vi "coincidenceImagenew.vi"(0 "notes 2":refnum<vi>) -> ()   [LabVIEW 2009]
uses:
  <vilib>/vision/NI_Vision_Development_Module.lvlib
panel:
  in  "notes":string
  in  "RGB/False":bool
  in  "Threshold":cluster{"max":u32, "min":u32}
  out "Photons":u32
  out "Spot No.":u8
  out "Ampel2":cluster{"RED":bool, "YELLOW":bool, "GREEN":bool}
  in  "spotsize (radius pixel)":u16=5 min=1 max=100
  in  "delayed channel":u8 max=7
  in  "length (µs)":dbl=10.0 format="%.2f"
  in  "lateral peaks":u32=2 min=2 max=10 step=2
  in  "center peak (µs)":dbl=0.6 format="%.2f"
  out "coincidence ratio":dbl format="%.2f"
  out "coincidence histogram":T1(graph)
  out "oval coordinates":i32[](array[numeric])
  out "Coordinates":i32[](array[numeric])
  in  "stop":bool
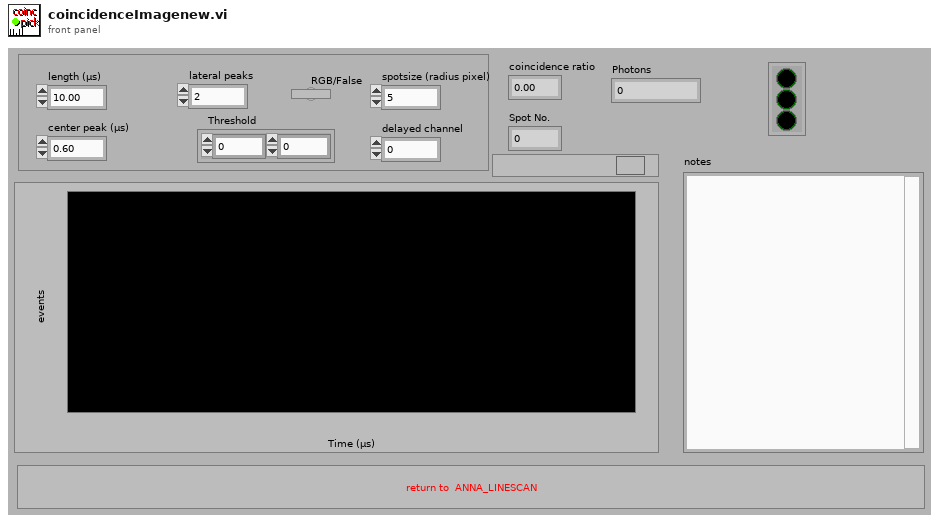
[diagram p1: front panel]
types:
  T1 = cluster{"Origin (ns)":dbl, "Offset (ns)":dbl, u32[]}
  T2 = cluster{"x0":i32, "y0":i32, "x1":i32, "y1":i32, "ovl std":i32[][]}
  T3 = enum16{"read/write", "read-only", "write-only", "write-only (truncate)"}
  T4 = typedef "IMAQ Image.ctl" = refnum<image>
  T5 = cluster{"origin (ns)":dbl, "offset (ns)":dbl, "histogram":u32[]}
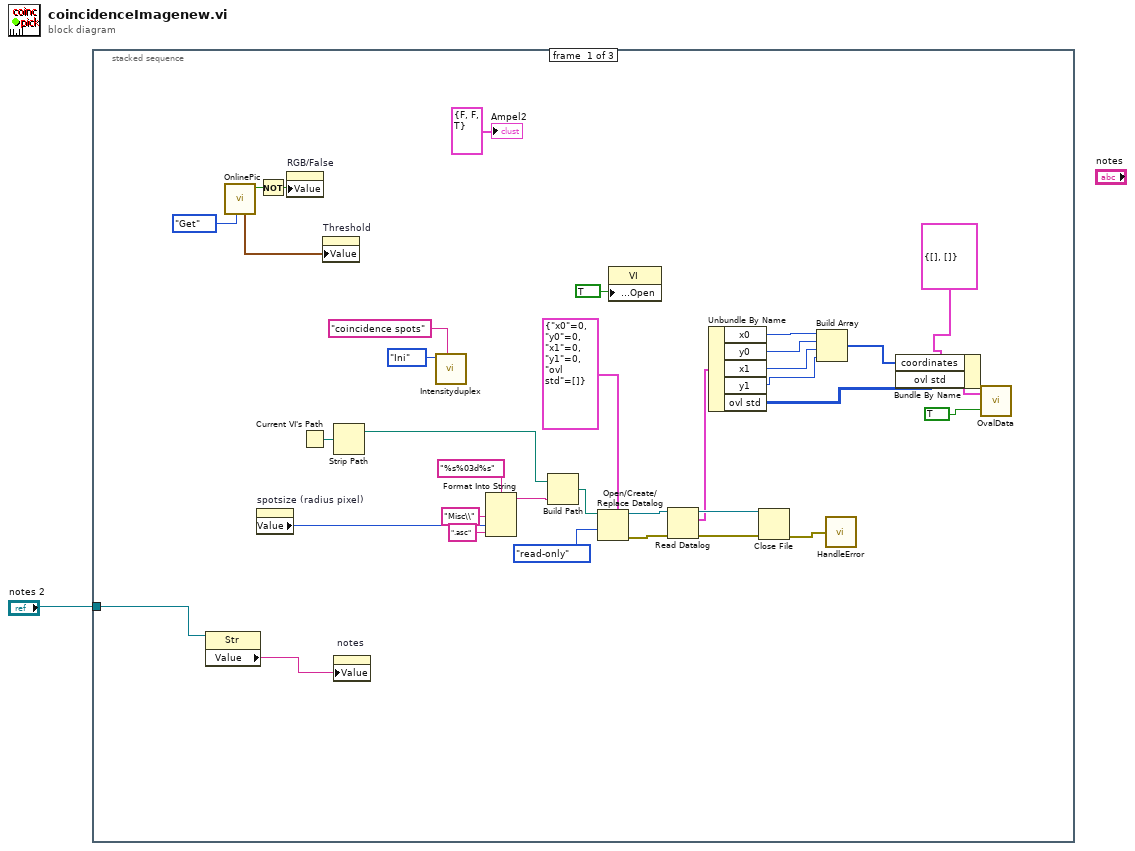
[diagram p0: block diagram]
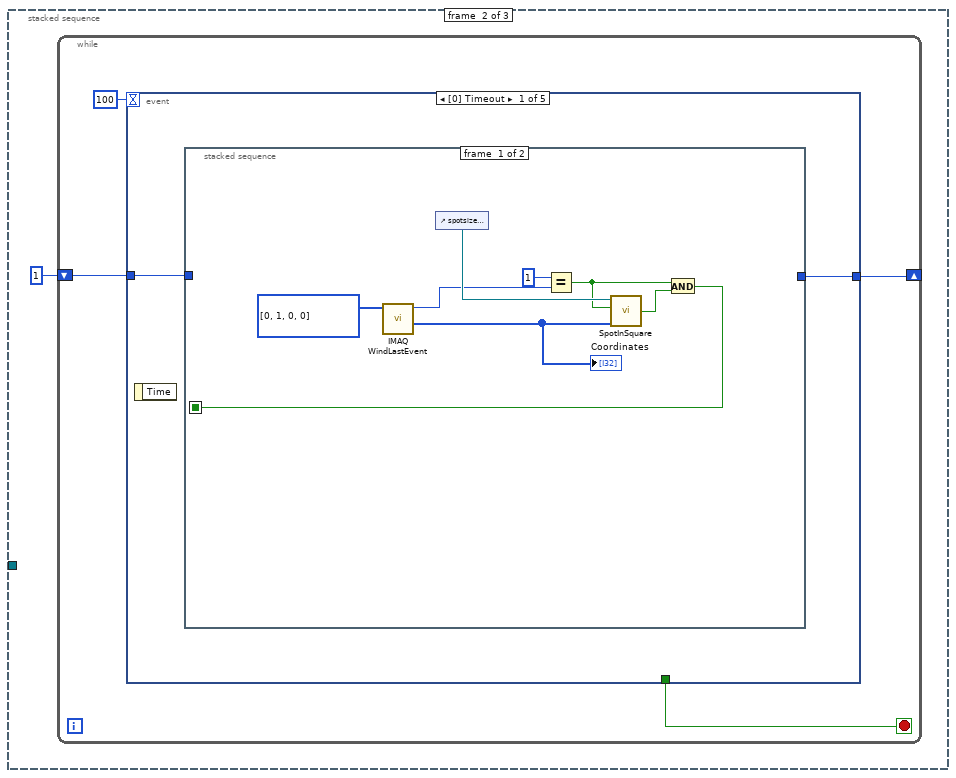
[diagram p2: hidden frame]
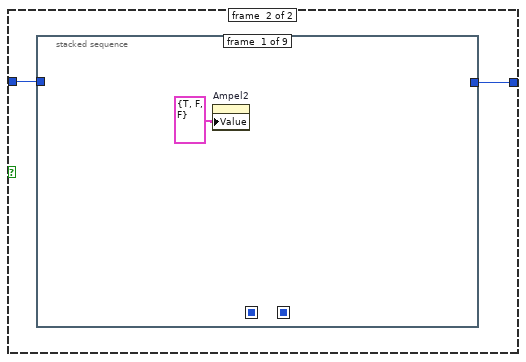
[diagram p4: hidden frame]
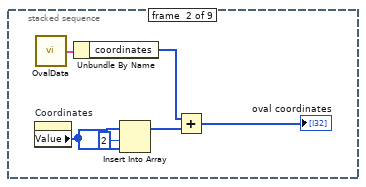
[diagram p5: hidden frame]
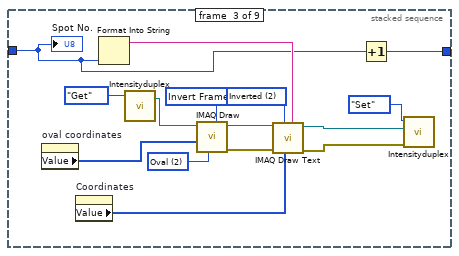
[diagram p6: hidden frame]
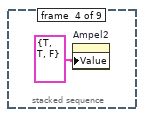
[diagram p7: hidden frame]
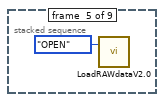
[diagram p8: hidden frame]
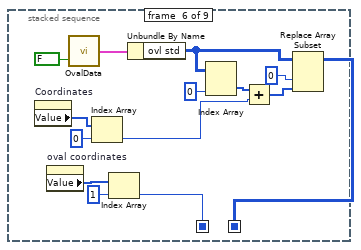
[diagram p9: hidden frame]
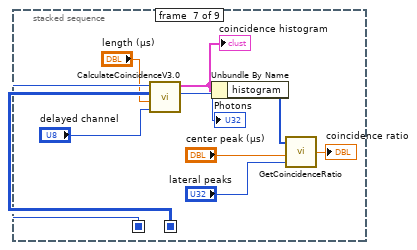
[diagram p10: hidden frame]
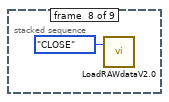
[diagram p11: hidden frame]
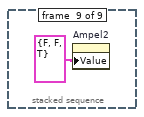
[diagram p12: hidden frame]
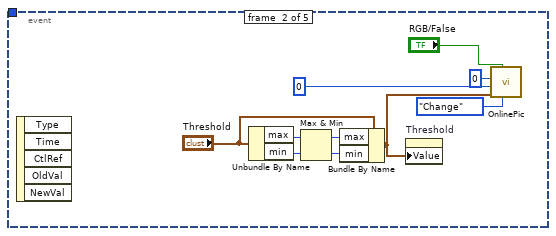
[diagram p13: hidden frame]
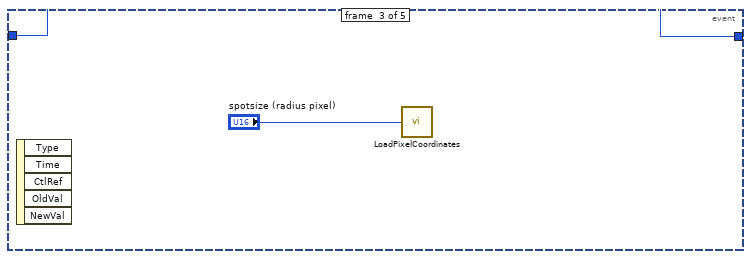
[diagram p14: hidden frame]
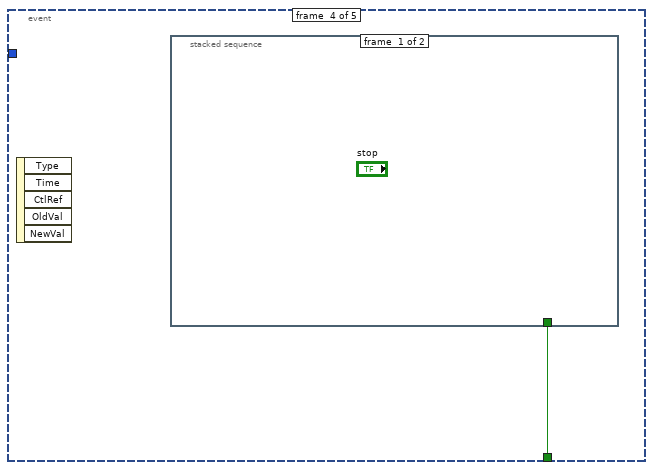
[diagram p15: hidden frame]
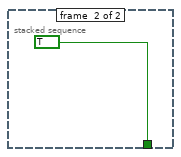
[diagram p16: hidden frame]
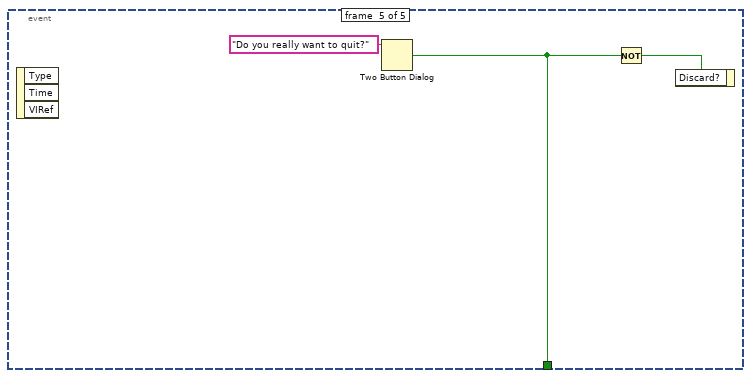
[diagram p17: hidden frame]
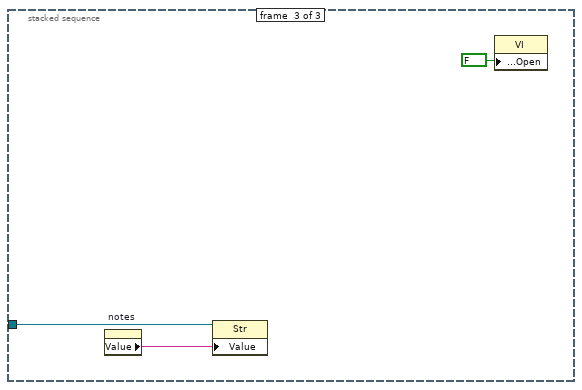
[diagram p18: hidden frame]
diagram:
  n1 = stacked-sequence {
    tunnel: "notes 2" -> [w3 _ w125]
    frame #0 {
      n2 = property class="Str"(reference=w3) -> ("Value"=w4:string)  [unwired: 1 in, 2 out]
      n3 = call "OnlinePic.vi"("action"=enum16{"Get", "Set", "Change", "ini"}."Get" ("Enum")) -> ("RGB/False out"=w28:bool, "Threshold (max) OUT"=w26:cluster{"max":u32, "min":u32})  [unwired: 6 in, 3 out]
      n4 = property on="spotsize (radius pixel)" class="Digital (strict)"() -> ("Value"=w32:u16)  [unwired: 2 in, 2 out]
      n5 = Not(x=w28) -> (.not. x?=w25:bool)
      n6 = property on="RGB/False" class="Boolean (strict)"("Value"=w25) -> ()  [unwired: 2 in, 2 out]
      n7 = Current VI's Path() -> (path=w17:path)
      n8 = property on="Threshold" class="Clust (strict)"("Value"=w26) -> ()  [unwired: 2 in, 2 out]
      n9 = Strip Path(path=w17) -> (stripped path=w16:path)  [unwired: 1 out]
      n10 = property on="notes" class="String"("Value"=w4) -> ()  [unwired: 2 in, 2 out]
      n11 = call "Intensityduplex.vi"("Enum"=enum16{"Ini", "Get", "Set", "Refresh", "dump"}."Ini", "title"="coincidence spots") -> ()  [unwired: 3 in, 2 out]
      n12 = Format Into String(format string="%s%03d%s", "Misc\\" ("input 1"), w32, ".asc" ("input 3")) -> (resulting string=w24:string)  [unwired: 2 in, 1 out]
      n13 = Build Path(base path=w16, name or relative path=w24) -> (appended path=w23:path)
      n14 = Open/Create/Replace Datalog(5:T2 {"x0"=0, "y0"=0, "x1"=0, "y1"=0, "ovl std"=[]} ("cluster"), 9:T3."read-only" ("open mode (0)"), 11:w23) -> (0:w22:errorcluster, 3:w20:refnum<k1>)  [unwired: 3 in, 1 out]
      n15 = property class="VI"("Front Panel Window:Open"=TRUE) -> ()  [unwired: 2 in, 2 out]
      n16 = Read Datalog(4:w22, 7:w20) -> (0:w21:errorcluster, 2:w13:T2, 3:w19:refnum<k1>)  [unwired: 1 in]
      n17 = Unbundle By Name(w13) -> ("x0"=w10:i32, "y0"=w9:i32, "x1"=w8:i32, "y1"=w7:i32, "ovl std"=w6:i32[][])
      n18 = Close File(refnum=w19, error in=w21) -> (error out=w2:errorcluster)  [unwired: 1 out]
      n19 = Build Array(w10, w9, w8, w7) -> (w5:i32[])
      n20 = call "HandleError.vi"("error in (no error)"=w2) -> ()
      n21 = Bundle By Name(cluster=cluster{"coordinates":i32[], "ovl std":i32[][]} {"coordinates"=[], "ovl std"=[]} ("data"), "coordinates"=w5, "ovl std"=w6) -> (w12:cluster{"coordinates":i32[], "ovl std":i32[][]})
      n22 = call "OvalData.vi"("changed?"=TRUE, "data 2"=w12) -> ()  [unwired: 1 out]
      "Ampel2" <- cluster{"RED":bool, "YELLOW":bool, "GREEN":bool} {"RED"=FALSE, "YELLOW"=FALSE, "GREEN"=TRUE} ("Ampel2")
    }
    frame #1 {
      n23 = while {
        shift-right: [w38] -> _
        shift-left: u8 1 -> [w39]
        stop <- w41 stop-if-true
        n24 = event shown="[0] Timeout" {
          selector: _ -> [_ _ _ _ _]
          dyn-events: _ -> [_ _ _ _ _]
          timeout: 100 -> [_ _ _ _ _]
          tunnel: [_ _ _ w120 w123] -> w41
          tunnel: w39 -> [w43 _ w119 _ _]
          tunnel: [w42 _ w119 _ _] -> w38
          event #0 {
            n25 = event-data() -> ()  [unwired: 1 in, 1 out]
            n26 = stacked-sequence {
              seq-local: [w44 _] -> [_ w52]
              tunnel: w43 -> [_ w54]
              tunnel: [_ w53] -> w42
              frame #0 {
                w51 = i32[] [0, 1, 0, 0] items=["No  event", "Click event", "Draw event", "Move event", "Size event", "Scroll event", "Activate event", "Close event", "Double click event"] ("Events list (all)")
                n27 = call "IMAQ WindLastEvent"("Events list (all)"=w51) -> ("Coordinates"=w50:i32[], "Event"=w48:i32)  [unwired: 5 in, 4 out]
                "Coordinates" <- w50
                n28 = control-ref of="spotsize (radius pixel)"() -> (w49:refnum<vi>)
                n29 = Equal?(x=1, y=w48) -> (x = y?=w45:bool)
                n30 = call "SpotInSquare.vi"("Coordinates"=w50, "event"=w45, "reference"=w49) -> ("Boolean"=w46:bool)  [unwired: 1 in]
                n31 = And(x=w45, y=w46) -> (x .and. y?=w44:bool)
              }
              frame #1 {
                n32 = case shown="False" w52 {
                  tunnel: w54 -> [w55 w57]
                  tunnel: [w55 w56] -> w53
                  frame #0 {
                  }
                  frame #1 {
                    n33 = stacked-sequence {
                      seq-local: [_ _ _ _ _ w89 _ _ _] -> [_ _ _ _ _ _ w105 _ _]
                      seq-local: [_ _ _ _ _ w84 _ _ _] -> [_ _ _ _ _ _ w104 _ _]
                      tunnel: w57 -> [_ _ w65 _ _ _ _ _ _]
                      tunnel: [_ _ w75 _ _ _ _ _ _] -> w56
                      frame #0 {
                        n34 = property on="Ampel2" class="Cluster (strict)"("Value"=cluster{"RED":bool, "YELLOW":bool, "GREEN":bool} {"RED"=TRUE, "YELLOW"=FALSE, "GREEN"=FALSE} ("Ampel2")) -> ()  [unwired: 2 in, 2 out]
                      }
                      frame #1 {
                        n35 = property on="Coordinates" class="Array (strict)"() -> ("Value"=w61:i32[])  [unwired: 2 in, 2 out]
                        n36 = call "OvalData.vi"() -> ("data"=w64:cluster{"coordinates":i32[], "ovl std":i32[][]})  [unwired: 2 in]
                        n37 = Unbundle By Name(w64) -> ("coordinates"=w62:i32[])
                        n38 = Insert Into Array(array=w61, index=2, new element=w61) -> (w59:i32[])
                        n39 = Add(x=w62, y=w59) -> (x+y=→"oval coordinates":i32[])
                      }
                      frame #2 {
                        w74 = 2 items=["White", "Black", "Inverted", "Black on White", "White on Black"] ("Color")
                        w78 = u16 2 items=["Line", "Rectangle", "Oval"] ("Shape to draw")
                        w79 = u16 2 items=["Frame", "Paint", "Invert Frame", "Invert Paint"] ("Draw Mode")
                        n40 = property on="oval coordinates" class="Array (strict)"() -> ("Value"=w69:i32[])  [unwired: 2 in, 2 out]
                        n41 = property on="Coordinates" class="Array (strict)"() -> ("Value"=w66:i32[])  [unwired: 2 in, 2 out]
                        n42 = Format Into String(w65) -> (resulting string=w76:string)  [unwired: 3 in, 1 out]
                        n43 = call "Intensityduplex.vi"("Enum"=enum16{"Ini", "Get", "Set", "Refresh"}."Get" ("command")) -> ("Image Duplicate (out)"=w77:T4)  [unwired: 4 in, 1 out]
                        n44 = call "IMAQ Draw"("Draw Mode"=w79, "Shape to draw"=w78, "Coordinates"=w69, "Image Src"=w77) -> ("error out"=w72:errorcluster, "Image Dst Out"=w73:T4)  [unwired: 6 in]
                        n45 = call "IMAQ Draw Text"("String"=w76, "Insertion Point"=w66, "Color"=w74, "error in (no error)"=w72, "Image Src"=w73) -> ("error out"=w71:errorcluster, "Image Dst Out"=w70:T4)  [unwired: 3 in, 2 out]
                        n46 = Increment(x=w65) -> (x+1=w75:u8)
                        n47 = call "Intensityduplex.vi"("Enum"=enum16{"Ini", "Get", "Set", "Refresh"}."Set" ("command"), "Image In"=w70, "error in"=w71) -> ()  [unwired: 2 in, 2 out]
                        "Spot No." <- w65
                      }
                      frame #3 {
                        n48 = property on="Ampel2" class="Cluster (strict)"("Value"=cluster{"RED":bool, "YELLOW":bool, "GREEN":bool} {"RED"=TRUE, "YELLOW"=TRUE, "GREEN"=FALSE} ("Ampel2")) -> ()  [unwired: 2 in, 2 out]
                      }
                      frame #4 {
                        n49 = call "LoadRAWdataV2.0.vi"("action"=enum16{"OPEN", "READ", "CLOSE"}."OPEN" ("Enum")) -> ()  [unwired: 1 in, 2 out]
                      }
                      frame #5 {
                        n50 = property on="Coordinates" class="Array (strict)"() -> ("Value"=w88:i32[])  [unwired: 2 in, 2 out]
                        n51 = property on="oval coordinates" class="Array (strict)"() -> ("Value"=w93:i32[])  [unwired: 2 in, 2 out]
                        n52 = call "OvalData.vi"("changed?"=FALSE) -> ("data"=w94:cluster{"coordinates":i32[], "ovl std":i32[][]})  [unwired: 1 in]
                        n53 = Index Array(array=w88, index=0) -> (element=w86:i32)
                        n54 = Index Array(array=w93, index=1) -> (element=w89:i32)
                        n55 = Unbundle By Name(w94) -> ("ovl std"=w85:i32[][])
                        n56 = Index Array(array=w85, index (col)=0 ("disabled index (col)")) -> (element=w90:i32[])  [unwired: 1 in]
                        n57 = Add(x=w90, y=w86) -> (x+y=w83:i32[])
                        n58 = Replace Array Subset(array=w85, new element=w83, index (col)=0 ("disabled index (col)")) -> (w84:i32[][])  [unwired: 1 in]
                      }
                      frame #6 {
                        n59 = call "CalculateCoincidenceV3.0.vi"("delayed channel"="delayed channel", "length (µs)"="length (µs)", "Pos Array"=w104, "starting y-point"=w105) -> ("Photons"=→"Photons":u32, "coincidence histogram"=w98:T5)  [unwired: 2 in]
                        "coincidence histogram" <- w98
                        n60 = Unbundle By Name(w98) -> ("histogram"=w100:u32[])
                        n61 = call "GetCoincidenceRatio.vi"("lateral peaks"="lateral peaks", "center peak (µs)"="center peak (µs)", "histogram"=w100) -> ("coincidence ratio"=→"coincidence ratio":dbl)
                      }
                      frame #7 {
                        n62 = call "LoadRAWdataV2.0.vi"("action"=enum16{"OPEN", "READ", "CLOSE"}."CLOSE" ("Enum")) -> ()  [unwired: 1 in, 2 out]
                      }
                      frame #8 {
                        n63 = property on="Ampel2" class="Cluster (strict)"("Value"=cluster{"RED":bool, "YELLOW":bool, "GREEN":bool} {"RED"=FALSE, "YELLOW"=FALSE, "GREEN"=TRUE} ("Ampel2")) -> ()  [unwired: 2 in, 2 out]
                      }
                    }
                  }
                }
              }
            }
          }
          event #1 {
            n64 = event-data() -> ()  [unwired: 1 in, 5 out]
            n65 = Unbundle By Name("Threshold") -> ("max"=w112:u32, "min"=w109:u32)
            n66 = Max & Min(x=w112, y=w109) -> (max(x,y)=w111:u32, min(x,y)=w110:u32)
            n67 = Bundle By Name(cluster="Threshold", "max"=w111, "min"=w110) -> (w108:cluster{"max":u32, "min":u32})
            n68 = property on="Threshold" class="Cluster (strict)"("Value"=w108) -> ()  [unwired: 2 in, 2 out]
            n69 = call "OnlinePic.vi"("action"=enum16{"Get", "Set", "Change", "ini"}."Change" ("Enum"), "RGB/False"="RGB/False", "Threshold (max)"=w108, "plane"=u16 0, "router channel"=u16 0) -> ()  [unwired: 2 in, 5 out]
          }
          event #2 {
            n70 = event-data() -> ()  [unwired: 1 in, 5 out]
            n71 = call "LoadPixelCoordinates.vi"("spotsize (radius pixel)"="spotsize (radius pixel)") -> ()
          }
          event #3 {
            n72 = event-data() -> ()  [unwired: 1 in, 5 out]
            n73 = stacked-sequence {
              tunnel: [_ TRUE] -> w120
              frame #0 {
              }
              frame #1 {
              }
            }
          }
          event #4 {
            n74 = event-data() -> ()  [unwired: 1 in, 3 out]
            n75 = Two Button Dialog(message="Do you really want to quit?") -> (T button?=w123:bool)  [unwired: 2 in]
            n76 = Not(x=w123) -> (.not. x?=w122:bool)
            n77 = event-data("Discard?"=w122) -> ()  [unwired: 1 in, 1 out]
          }
        }
      }
    }
    frame #2 {
      n78 = property on="notes" class="String"() -> ("Value"=w126:string)  [unwired: 2 in, 2 out]
      n79 = property class="Str"(reference=w125, "Value"=w126) -> ()  [unwired: 1 in, 2 out]
      n80 = property class="VI"("Front Panel Window:Open"=FALSE) -> ()  [unwired: 2 in, 2 out]
    }
  }
